vi "Start ILC.vi"(8 "error in (no error)":errorcluster, 11 "Model in":refnum<class "Model.lvclass">) -> (0 "error out":errorcluster, 3 "Model out":refnum<class "Model.lvclass">)   [LabVIEW 2016, in "Model.lvclass"]
uses:
  Model.lvclass
  Model.lvclass/Model.ctl
  Modbus/DesktopModbus/DesktopModbus.lvclass
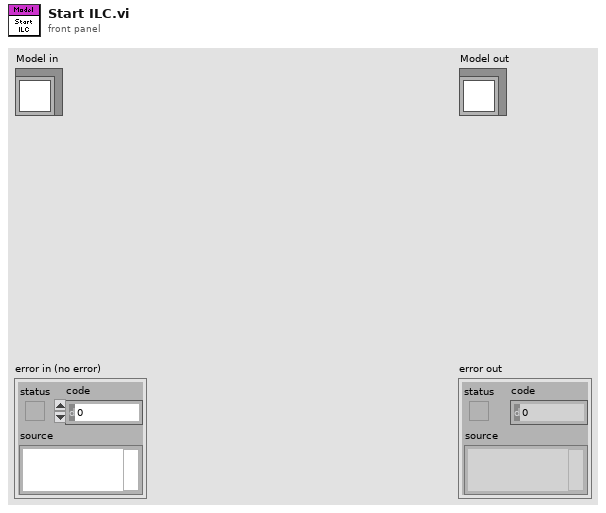
[diagram p1: front panel]
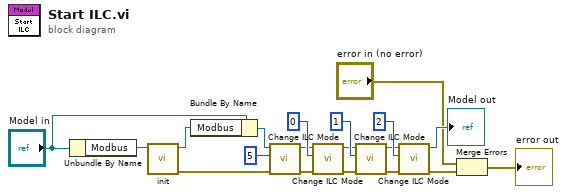
[diagram p0: block diagram]
diagram:
  n1 = Unbundle By Name("Model in") -> ("Modbus"=w5:refnum<class "DesktopModbus.lvclass">)
  n2 = call "init.vi"("DesktopModbus in"=w5) -> ("error out"=w3:errorcluster, "DesktopModbus out"=w4:refnum<class "DesktopModbus.lvclass">)  [unwired: 9 in]
  n3 = Bundle By Name(cluster="Model in", "Modbus"=w4) -> (w6:refnum<class "Model.lvclass">)
  n4 = call "Change ILC Mode.vi"("error in (no error)"=w3, "Mode"=u16 5, "Model in"=w6) -> ("error out"=w18:errorcluster, "Model out"=w13:refnum<class "Model.lvclass">)  [unwired: 7 in]
  n5 = call "Change ILC Mode.vi"("error in (no error)"=w18, "Mode"=u16 0, "Model in"=w13) -> ("error out"=w1:errorcluster, "Model out"=w2:refnum<class "Model.lvclass">)  [unwired: 7 in]
  n6 = call "Change ILC Mode.vi"("error in (no error)"=w1, "Mode"=u16 1, "Model in"=w2) -> ("error out"=w19:errorcluster, "Model out"=w16:refnum<class "Model.lvclass">)  [unwired: 7 in]
  n7 = call "Change ILC Mode.vi"("error in (no error)"=w19, "Mode"=u16 2, "Model in"=w16) -> ("error out"=w10:errorcluster, "Model out"=→"Model out":refnum<class "Model.lvclass">)  [unwired: 7 in]
  n8 = Merge Errors("error in (no error)", w10) -> (→"error out":errorcluster)
